vi "remote-control.vi"() -> ()   [LabVIEW 2009]
panel:
  in  "command (12bit)":u16 max=4095 format="%.0x"
  in  "IRSND USB Device":refnum<visa-resource-name>
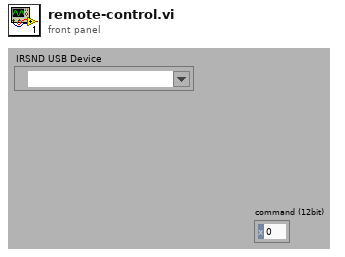
[diagram p1: front panel]
types:
  T1 = cluster{"protocol":u8, " address":u16, " command":u16, " flags":u8}
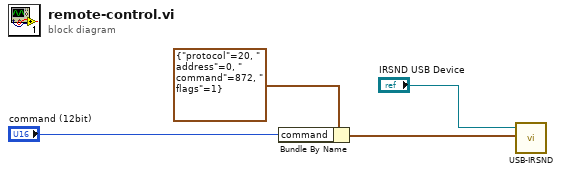
[diagram p0: block diagram]
diagram:
  n1 = Bundle By Name(cluster=T1 {"protocol"=20, " address"=0, " command"=872, " flags"=1} ("irmp_data"), "command"="command (12bit)") -> (w1:T1)
  n2 = call "USB-IRSND.vi"("irmp_data"=w1, "IRSND USB Device"="IRSND USB Device") -> ()  [unwired: 2 in, 1 out]
